vi "ShowAll.vi"(7 "Tab Control 2":enum32{"RT Monitor", "IV Monitor"}(tab), 10 "Bias":waveform(dbl), 11 "Traces":waveform(dbl)[](array[waveform])) -> ()   [LabVIEW 2024]
panel:
  out "Waveform Chart 7":waveform(dbl)(graph)
  out "Waveform Chart 6":waveform(dbl)(graph)
  out "Waveform Chart 5":waveform(dbl)(graph)
  out "Waveform Chart 4":waveform(dbl)(graph)
  out "Waveform Chart 3":waveform(dbl)(graph)
  out "Waveform Chart 2":waveform(dbl)(graph)
  out "Waveform Chart":waveform(dbl)(graph)
  out "Waveform Chart":waveform(dbl)(graph)
  out "2d array of graphs":cluster{"XY Graph":cluster{dbl, dbl}[]}[][](array[cluster])
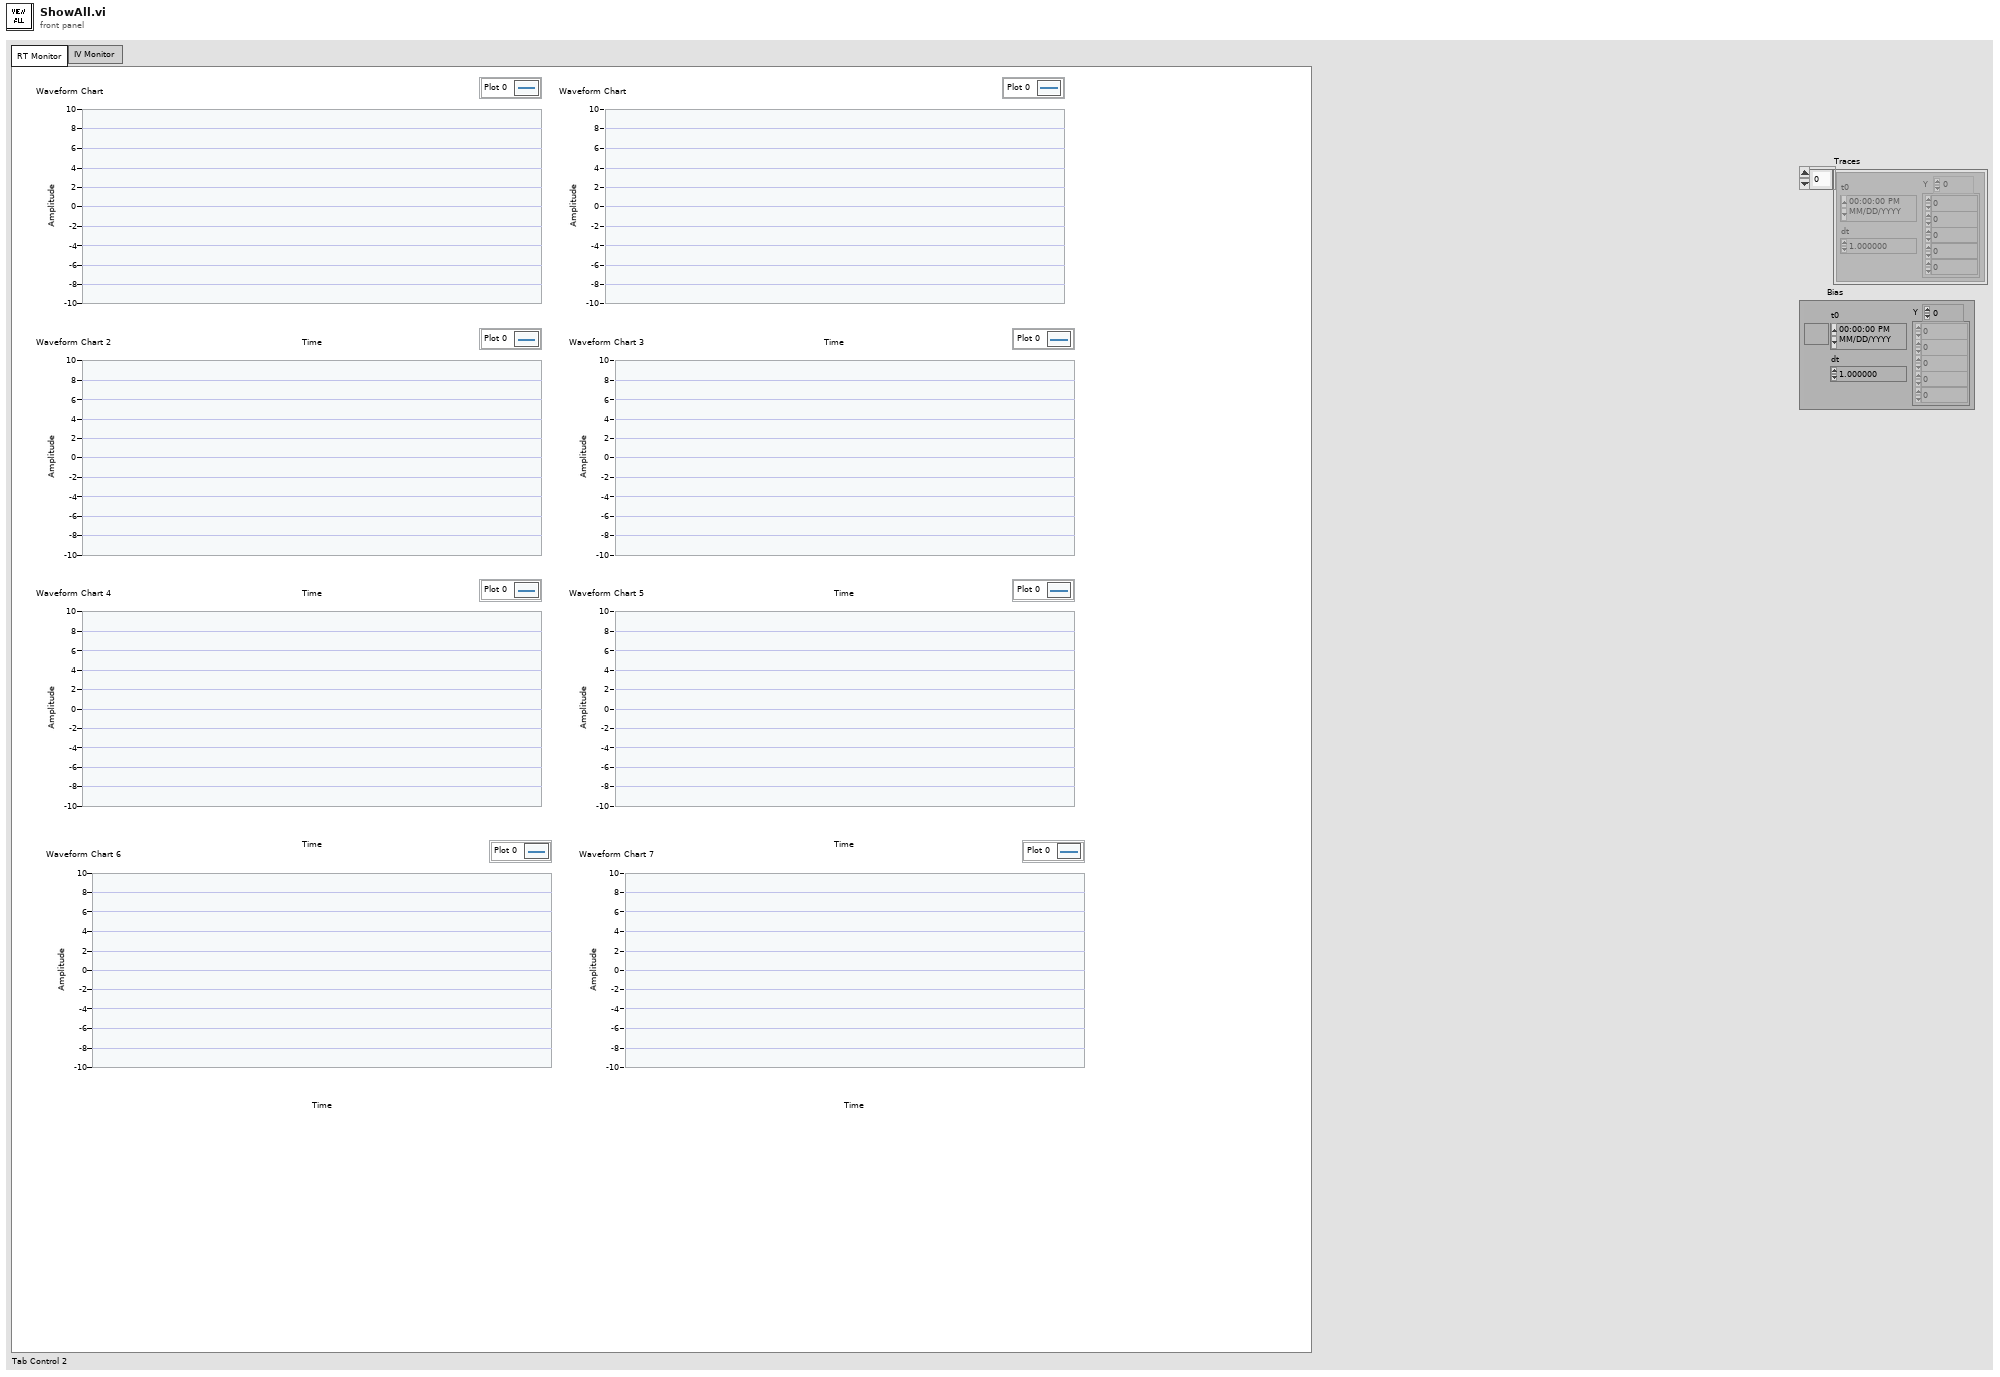
[diagram p1: front panel]
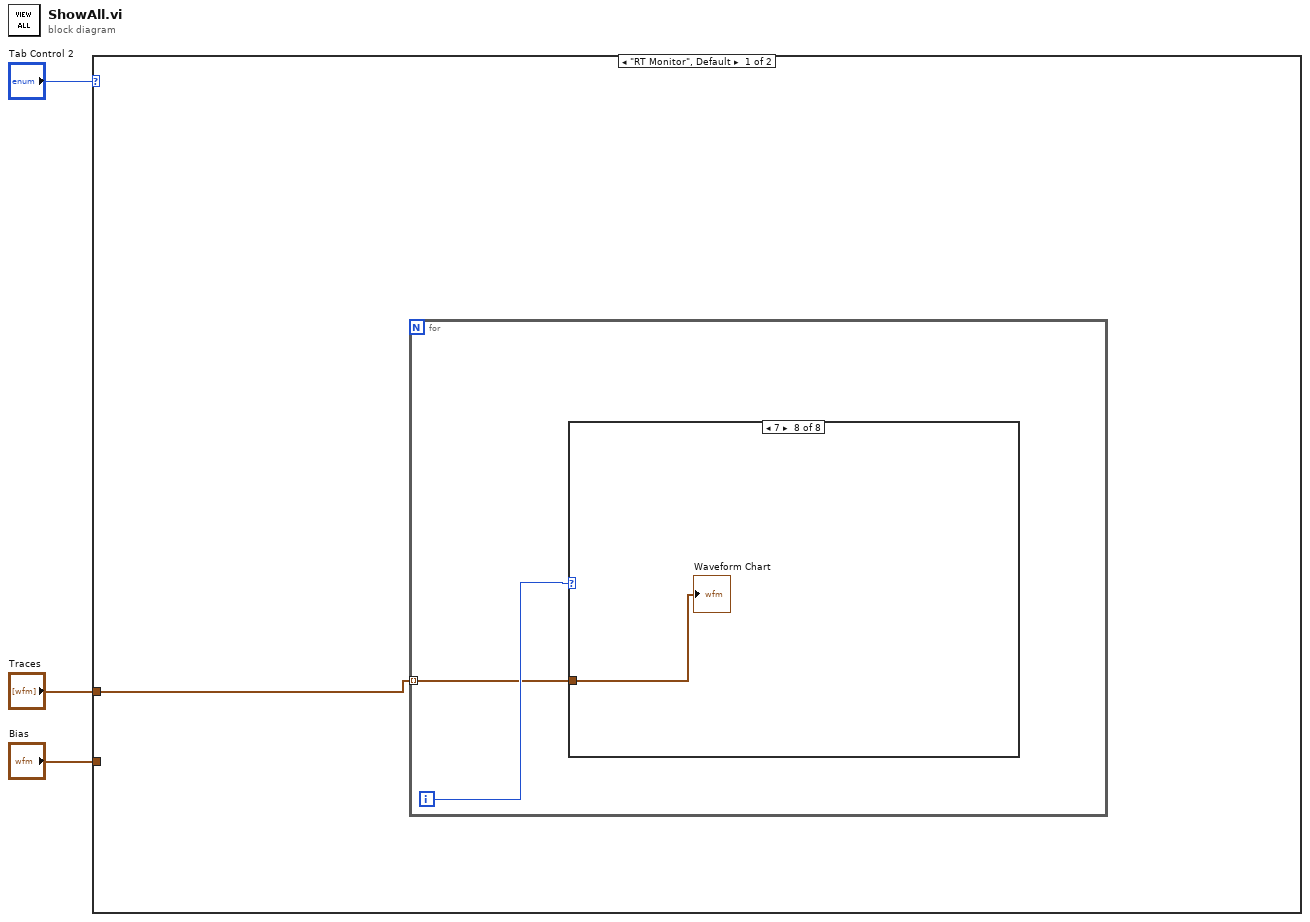
[diagram p0: block diagram]
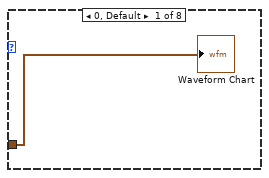
[diagram p2: hidden frame]
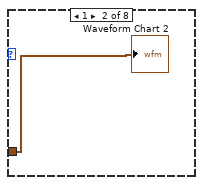
[diagram p3: hidden frame]
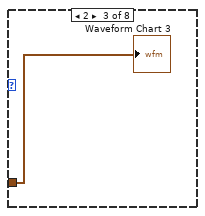
[diagram p4: hidden frame]
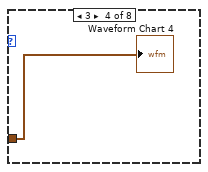
[diagram p5: hidden frame]
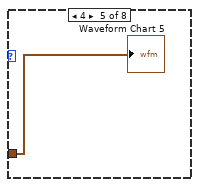
[diagram p6: hidden frame]
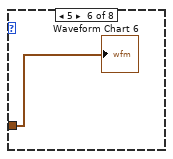
[diagram p7: hidden frame]
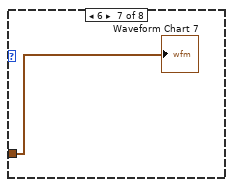
[diagram p8: hidden frame]
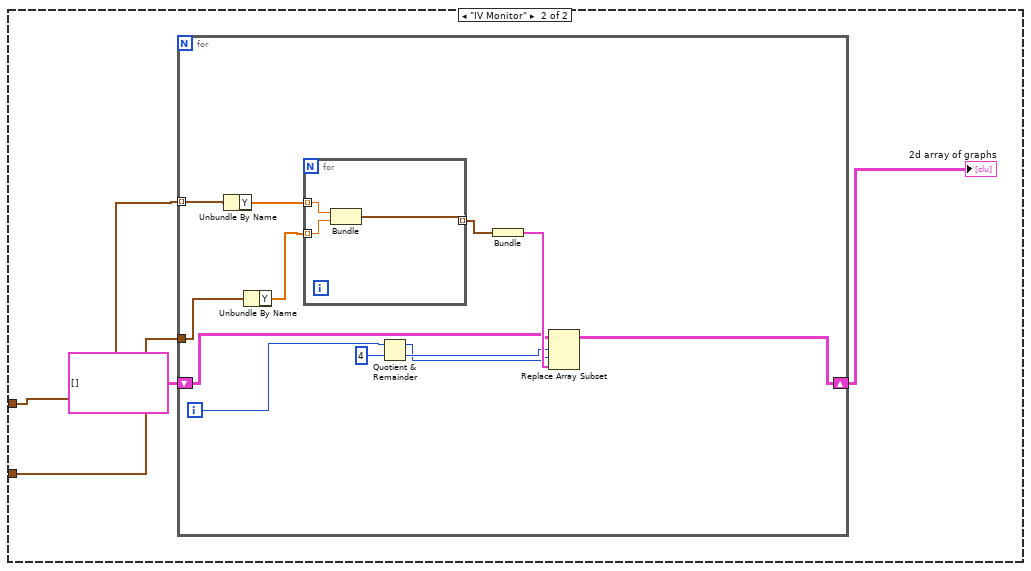
[diagram p9: hidden frame]
diagram:
  n1 = case shown="\"RT Monitor\", Default" "Tab Control 2" {
    tunnel: "Traces" -> [w4 w18]
    tunnel: "Bias" -> [_ w17]
    frame "RT Monitor", Default {
      n2 = for {
        tunnel: w4 -> [w5] mode=indexing
        i -> [w6]
        n3 = case shown="7" w6 {
          tunnel: w5 -> [w7 w8 w9 w10 w11 w12 w13 w14]
          frame 0, Default {
            "Waveform Chart" <- w7
          }
          frame 1 {
            "Waveform Chart 2" <- w8
          }
          frame 2 {
            "Waveform Chart 3" <- w9
          }
          frame 3 {
            "Waveform Chart 4" <- w10
          }
          frame 4 {
            "Waveform Chart 5" <- w11
          }
          frame 5 {
            "Waveform Chart 6" <- w12
          }
          frame 6 {
            "Waveform Chart 7" <- w13
          }
          frame 7 {
            "Waveform Chart" <- w14
          }
        }
      }
    }
    frame "IV Monitor" {
      n4 = for {
        tunnel: w18 -> [w30] mode=indexing
        tunnel: w17 -> [w29]
        shift-right: [w21] -> w15
        shift-left: cluster{cluster{dbl, dbl}[]}[][] [] -> [w22]
        i -> [w25]
        n5 = Unbundle By Name(w30) -> ("Y"=w28:dbl[])
        n6 = Unbundle By Name(w29) -> ("Y"=w27:dbl[])
        n7 = for {
          tunnel: w28 -> [w33] mode=indexing
          tunnel: w27 -> [w32] mode=indexing
          tunnel: [w31] -> w26 mode=indexing
          n8 = Bundle(w33, w32) -> (w31:cluster{dbl, dbl})  [unwired: 1 in]
        }
        n9 = Quotient & Remainder(x=w25, y=4) -> (x-y*floor(x/y)=w19:i32, floor(x/y)=w20:i32)
        n10 = Bundle(w26) -> (w23:cluster{cluster{dbl, dbl}[]})  [unwired: 1 in]
        n11 = Replace Array Subset(array=w22, new element=w23, index (row)=w20, index (col)=w19) -> (w21:cluster{cluster{dbl, dbl}[]}[][])
      }
      "2d array of graphs" <- w15
    }
  }
